vi "Contour Controls Show Hide.vi"(5 "Contour Mode":enum16{"Contour", "Contour with surface"}(ring) caption="Contour mode", 6 "Line Color Ref":refnum<vi>, 7 "Level Mode":enum16{"Levels", "Interval", "Level List"}(ring), 8 "error in (no error)":errorcluster, 9 "Level List Ref":refnum<vi>, 10 "Interval Ref":refnum<vi>, 11 "Levels Ref":refnum<vi>) -> (0 "error out":errorcluster)   [LabVIEW 2020, in "3D Contour.lvclass"]
uses:
  <vilib>/Math Plots/3D Math Plots/3D Contour/3D Contour/3D Contour.lvclass
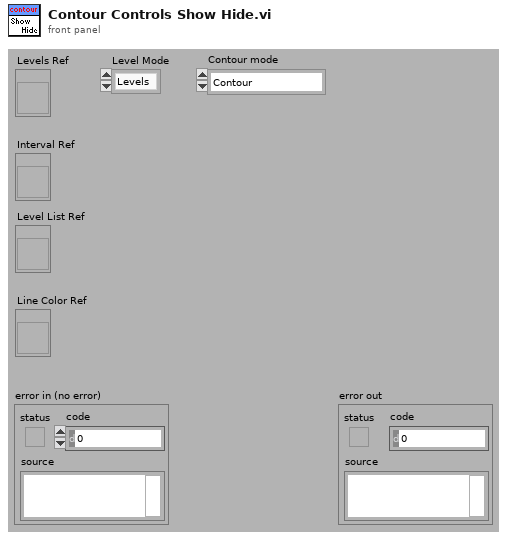
[diagram p1: front panel]
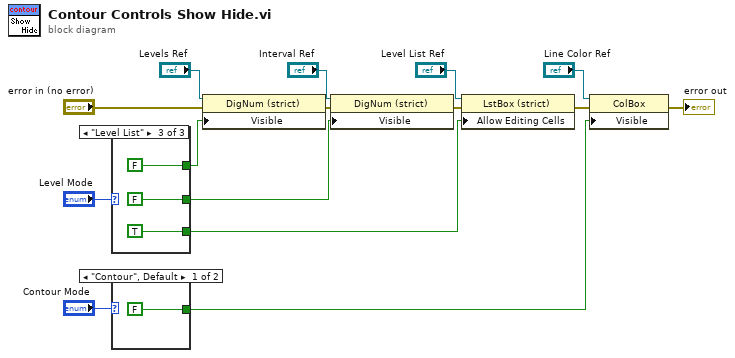
[diagram p0: block diagram]
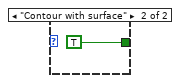
[diagram p2: hidden frame]
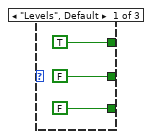
[diagram p3: hidden frame]
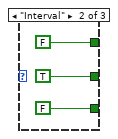
[diagram p4: hidden frame]
diagram:
  n1 = case shown="\"Level List\"" "Level Mode" {
    tunnel: [TRUE FALSE FALSE] -> w9
    tunnel: [FALSE TRUE FALSE] -> w8
    tunnel: [FALSE FALSE TRUE] -> w7
    frame "Levels", Default {
    }
    frame "Interval" {
    }
    frame "Level List" {
    }
  }
  n2 = case shown="\"Contour\", Default" "Contour Mode" {
    tunnel: [FALSE TRUE] -> w3
    frame "Contour", Default {
    }
    frame "Contour with surface" {
    }
  }
  n3 = property on="Property Node" class="DigNum (strict)"(reference="Levels Ref", error in="error in (no error)", "Visible"=w9) -> (error out=w14:errorcluster)  [unwired: 1 out]
  n4 = property on="Property Node" class="DigNum (strict)"(reference="Interval Ref", error in=w14, "Visible"=w8) -> (error out=w15:errorcluster)  [unwired: 1 out]
  n5 = property on="Property Node" class="LstBox (strict)"(reference="Level List Ref", error in=w15, "Allow Editing Cells"=w7) -> (error out=w5:errorcluster)  [unwired: 1 out]
  n6 = property on="Property Node" class="ColBox"(reference="Line Color Ref", error in=w5, "Visible"=w3) -> (error out=→"error out":errorcluster)  [unwired: 1 out]
